vi "Generador_Entorno_2(SubVi).vi"(6 "Archivos_Constantes":u16, 8 "Entrada de Texto":string[](array[string]), 9 "Objetos":path=path "C:/Users/LuisFernando/Documents/UPIITA/8vo semestre/Instrumentacion Virtual Aplicada/Solidworks/2_Ejes_Figuras/Figuras", 10 "Mundo":path=path "C:/Users/LuisFernando/Documents/UPIITA/8vo semestre/Instrumentacion Virtual Aplicada/Solidworks/2_Ejes_Figuras/Mundo.wrl", 11 "Cluster":cluster{"Translación":dbl[][]}={"Translación"=[[1.0, 1.0, 0.0], [0.0, 0.0, 0.0], [0.0, 0.0, 0.0]]}) -> (3 "3D Picture":refnum<vi>(3d-picture))   [LabVIEW 2017]
uses:
  <vilib>/picture/3D Picture Control/NI_3D Picture Control.lvlib
panel:
  out "Archivos":i32
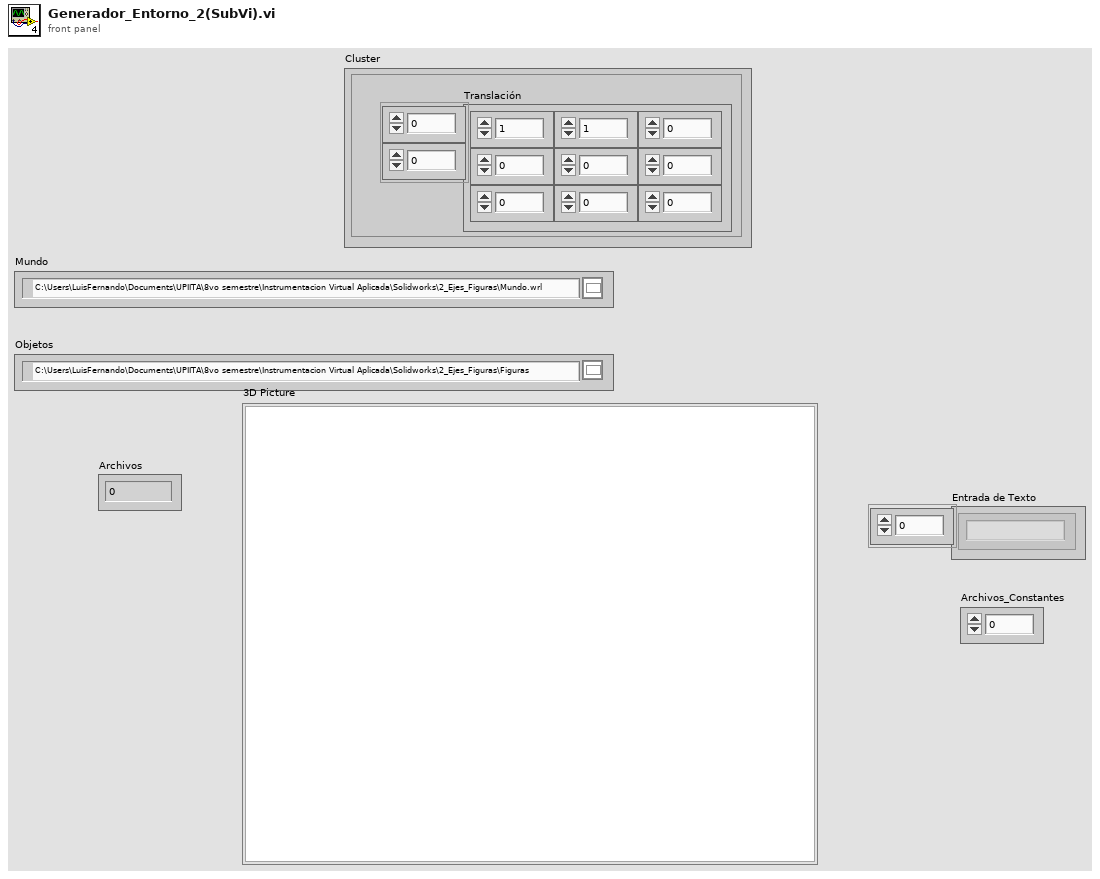
[diagram p1: front panel]
types:
  T1 = cluster{"Escala":dbl[][], "Translación":dbl[][], "Rotación":dbl[][]}
  T2 = enum16{"open", "replace", "create", "open or create", "replace or create", "replace or create with confirmation"}
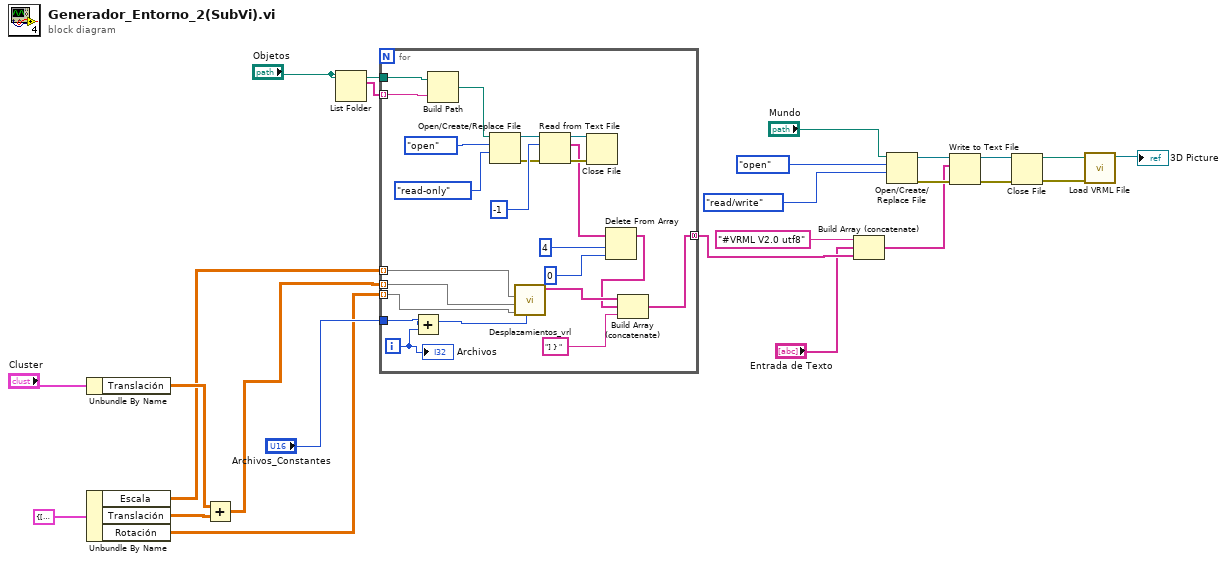
[diagram p0: block diagram]
diagram:
  n1 = Unbundle By Name("Cluster") -> ("Translación"=w4:dbl[][])
  n2 = Unbundle By Name(T1 {"Escala"=[[0.1, 0.1, 0.1], [0.3, 0.3, 0.3], [1.0, 1.0, 1.0]], "Translación"=[[0.0, 0.7999999999999998, 0.0], [0.0, 0.0, 0.0], [0.0, 0.0, 0.0]], "Rotación"=[[1.0, 0.0, 0.0, 0.0], [1.0, 0.0, 0.0, 0.0], [1.0, 0.0, 0.0, 0.0]]} ("Cluster_Moviles")) -> ("Escala"=w2:dbl[][], "Translación"=w5:dbl[][], "Rotación"=w1:dbl[][])
  n3 = Add(x=w4, y=w5) -> (x+y=w3:dbl[][])
  n4 = List Folder(path="Objetos") -> (filenames=w17:string[])  [unwired: 3 in, 3 out]
  n5 = for {
    tunnel: w17 -> [w47] mode=indexing
    tunnel: "Objetos" -> [w46]
    tunnel: [w33] -> w9 mode=concatenating
    tunnel: w3 -> [w34] mode=indexing
    tunnel: "Archivos_Constantes" -> [w27]
    tunnel: w2 -> [w26] mode=indexing
    tunnel: w1 -> [w25] mode=indexing
    i -> [w28]
    n6 = Add(x=w27, y=w28) -> (x+y=w29:i32)
    n7 = Build Path(base path=w46, name or relative path=w47) -> (appended path=w45:path)
    n8 = Open/Create/Replace File(file path (use dialog)=w45, operation (0:open)=T2."open", access (0:read/write)=enum16{"read/write", "read-only", "write-only"}."read-only") -> (refnum out=w42:refnum<file>, error out=w40:errorcluster)  [unwired: 3 in, 1 out]
    n9 = call "Desplazamientos_vrl.vi"("Indice"=w29, "Rotacion"=w25, "Translacion"=w34, "Escala"=w26) -> ("Salida"=w31:string[])  [unwired: 7 in]
    n10 = Read from Text File(file (use dialog)=w42, count=-1, error in=w40) -> (refnum out=w38:refnum<file>, text=w35:string[], error out=w39:errorcluster)  [unwired: 1 in, 1 out]
    n11 = Close File(refnum=w38, error in=w39) -> ()  [unwired: 2 out]
    n12 = Delete From Array(array=w35, length=4, index=0) -> (array with subset deleted=w30:string[])  [unwired: 1 out]
    n13 = Build Array (concatenate)(w31, w30, "] } ") -> (w33:string[])
    "Archivos" <- w28
  }
  n14 = Build Array (concatenate)("#VRML V2.0 utf8", "Entrada de Texto", w9) -> (w12:string[])
  n15 = Open/Create/Replace File(file path (use dialog)="Mundo", operation (0:open)=T2."open", access (0:read/write)=enum16{"read/write", "read-only", "write-only"}."read/write") -> (refnum out=w21:refnum<file>, error out=w20:errorcluster)  [unwired: 3 in, 1 out]
  n16 = Write to Text File(file (use dialog)=w21, text=w12, error in=w20) -> (refnum out=w18:refnum<file>, error out=w19:errorcluster)  [unwired: 1 in, 1 out]
  n17 = Close File(refnum=w18, error in=w19) -> (path=w15:path, error out=w14:errorcluster)
  n18 = call <vilib>:"Load VRML File.vi"("error in"=w14, "Path"=w15) -> ("Scene:Read Scene File"=→"3D Picture":refnum<vi>)  [unwired: 8 in, 1 out]
